vi "Init from Node-ID.vi"(7 "Function code":T1=12 items=["EMCY"=1, "PDO1 (tx)"=3, "PDO1 (rx)"=4, "PDO2 (tx)"=5, "PDO2 (rx)"=6, "PDO3 (tx)"=7, "PDO3 (rx)"=8, "PDO4 (tx)"=9, "PDO4 (rx)"=10, "SDO (tx)"=11, "SDO (rx)"=12, "NMT error control"=14], 9 "Data":u8[](array[numeric]) format="%.0x", 10 "Node-ID":u8, 11 "CANopen Message in":refnum<class "CANopen Message.lvclass">) -> (3 "CANopen Message out":refnum<class "CANopen Message.lvclass">)   [LabVIEW 2024, in "CANopen Master.lvlib" / "CANopen Message.lvclass"]
uses:
  CANopen Message.lvclass
  CANopen Message.lvclass/CANopen Message.ctl
  CANopen/FunctionCode.ctl
  CANopen Master.lvlib
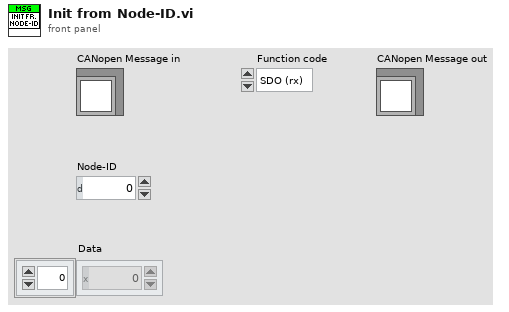
[diagram p1: front panel]
types:
  T1 = typedef "CANopen Master.lvlib/FunctionCode.ctl" = u16
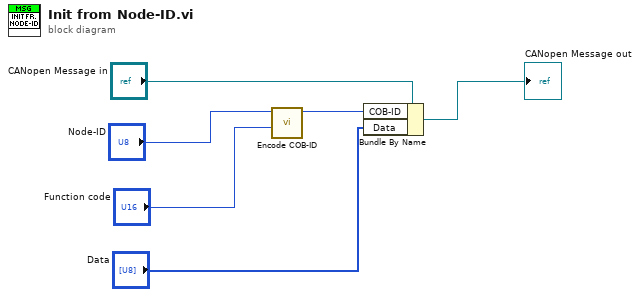
[diagram p0: block diagram]
diagram:
  n1 = call "Encode COB-ID.vi"("Function code"="Function code", "Node-ID"="Node-ID") -> ("COD-ID"=w2:u32)  [unwired: 9 in]
  n2 = Bundle By Name(cluster="CANopen Message in", "COB-ID"=w2, "Data"="Data") -> (→"CANopen Message out":refnum<class "CANopen Message.lvclass">)
